vi "auto_ctrl_valve_periodic.vi"(4 "auto_ctrl_per":bool=TRUE caption="Periodic\nControl", 6 "ref_sp_turn":refnum<vi>, 7 "counter_in":u32) -> (5 "counter_out":u32)   [LabVIEW 2019]
doc: "This example demonstrates how to simulate a general PID controller."
panel:
  in  "turn_close":dbl format="%.1f"
  in  "count_to_close":u32=150
  in  "count_to_open":u32=120
  in  "turn_open":dbl=3.0 format="%.1f"
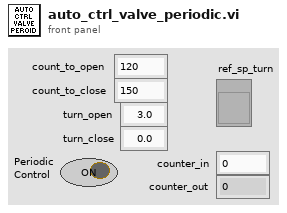
[diagram p1: front panel]
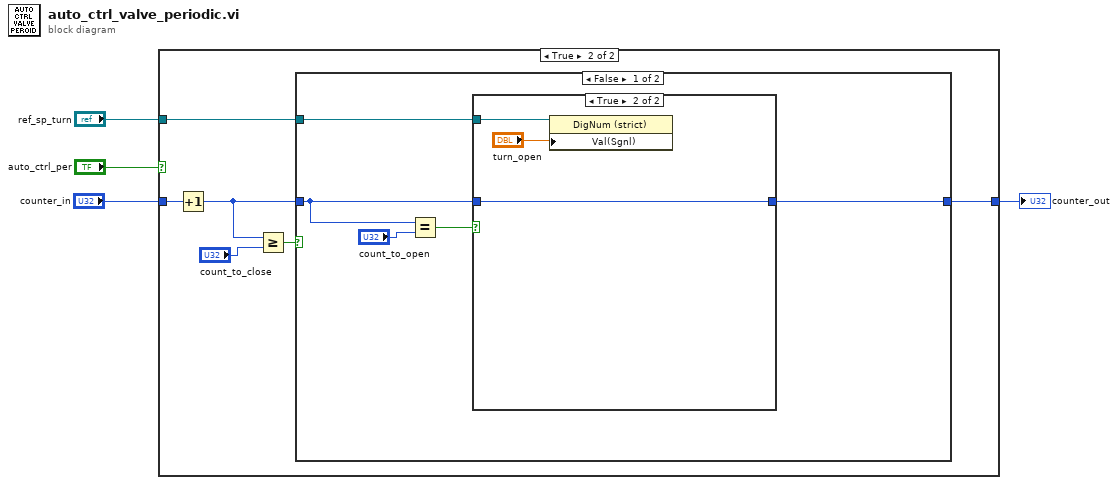
[diagram p0: block diagram]
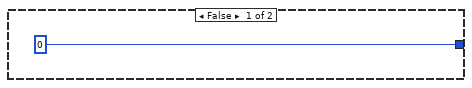
[diagram p2: hidden frame]
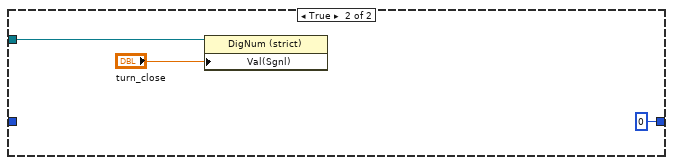
[diagram p4: hidden frame]
diagram:
  n1 = case shown="True" "auto_ctrl_per" {
    tunnel: [u32 0 ("alarm_status") w11] -> w2
    tunnel: "ref_sp_turn" -> [_ w10]
    tunnel: "counter_in" -> [_ w8]
    frame False {
    }
    frame True {
      n2 = Increment(x=w8) -> (x+1=w6:u32)
      n3 = Greater Or Equal?(x=w6, y="count_to_close") -> (x >= y?=w9:bool)
      n4 = case shown="False" w9 {
        tunnel: [w12 u32 0 ("alarm_status")] -> w11
        tunnel: w10 -> [w14 w23]
        tunnel: w6 -> [w13 _]
        frame False {
          n5 = Equal?(x=w13, y="count_to_open") -> (x = y?=w15:bool)
          n6 = case shown="True" w15 {
            tunnel: w14 -> [_ w20]
            tunnel: w13 -> [w17 w18]
            tunnel: [w17 w18] -> w12
            frame False {
            }
            frame True {
              n7 = property class="DigNum (strict)"(reference=w20, "Val(Sgnl)"="turn_open") -> ()  [unwired: 1 in, 2 out]
            }
          }
        }
        frame True {
          n8 = property class="DigNum (strict)"(reference=w23, "Val(Sgnl)"="turn_close") -> ()  [unwired: 1 in, 2 out]
        }
      }
    }
  }
  "counter_out" <- w2
